vi "RS232RxDataFIFO.vi"   [LabVIEW 2016]
uses:
  <vilib>/rvi/Emulation/niFpgaGetClockAttributes.vi
  <vilib>/rvi/Emulation/niFpgaSctlEmulationGetInTimedLoop.vi
  <vilib>/rvi/Emulation/niFpgaEmulationReportErrorSimple.vi
  <vilib>/rvi/Emulation/niFpgaEmulationIsFPGAContextNoSignature.vi
  <vilib>/rvi/FIFO/Fifo_Resource/nirvififoEmulationSetSize.vi
  <vilib>/rvi/DataTransferAndStorage/Container/Common/niFpgaContainerGetUniqueNameForEmu.vi
  <vilib>/rvi/FIFO/Fifo_Resource/nirviFifoEmulationQueueMgr.vi
  <instcachedir>/0/nirviFifoEmulationQueueMgr_E5CAEC123FF24DC58D834DCA3CDAA9B5.lvgen/nirviFifoEmulationQueueMgr_E5CAEC123FF24DC58D834DCA3CDAA9B5_009.vi
  <vilib>/rvi/Emulation/niFpgaProcessEmulError.vi
  <vilib>/rvi/interface/RandomDataEmulation/niFpgaRandomDataHandleErrors.vi
  <vilib>/rvi/errors/niFpgaSetErrorForExecOnDevCompSimple.vi
  <vilib>/rvi/eio/common/nirviEmuReportErrorAndStop.vi
  <vilib>/Utility/error.llb/Clear Errors.vi
  <vilib>/rvi/FIFO/Fifo_Resource/nirvififoEmulationCreateLock.vi
  <vilib>/rvi/FIFO/Fifo_Resource/nirvififoEmulationObtainLock.vi
  <vilib>/rvi/FIFO/Fifo_Resource/nirvififoEmulationReleaseLock.vi
  <vilib>/rvi/occurrence/nirviWaitOnOccurrenceBase.vi
  <vilib>/rvi/errors/nirviReportUnexpectedCaseInternalError.vi
  <vilib>/rvi/errors/nirviReportUnexpectedCaseInternalError (U32).vi
  <vilib>/rvi/Emulation/niFpgaCriticalErrorInLSC.vi
  <vilib>/rvi/DataTransferAndStorage/Container/XNode/niFpgaContainer.xnode
  <vilib>/rvi/FIFO/Fifo_Resource/nirvififoEmulationGetNumberOfElementsToRead.vi
  <vilib>/rvi/interface/RandomDataEmulation/nirviRandomDataFpgaReadWriteTemplate.vi
  <vilib>/rvi/FIFO/Fifo_Resource/nirvififoEmulationRead.vi
  Common_FPGA_FIFO/FPGAFIFO.lvlib
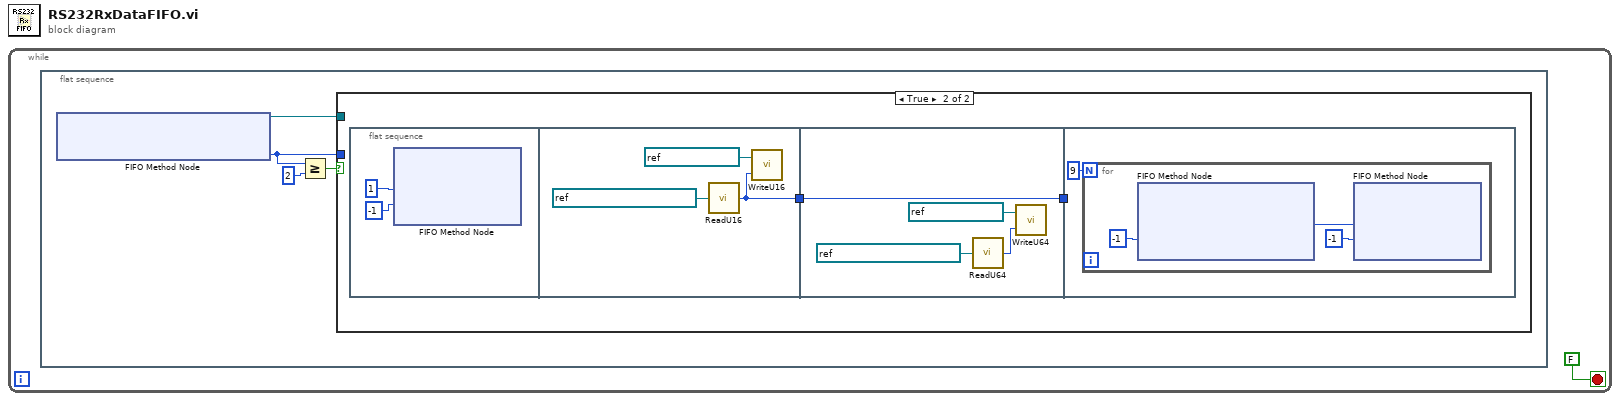
[diagram p0: block diagram]
diagram:
  n1 = while {
    stop <- FALSE stop-if-true
    n2 = flat-sequence {
      frame #0 {
        n3 = xnode ("FIFO Method Node")() -> ("Number of Elements to Read"=w2:u32, "FIFO Out"=w3:refnum<k21>)  [unwired: 1 in]
        n4 = Greater Or Equal?(x=w2, y=u32 2) -> (x >= y?=w4:bool)
        n5 = case shown="True" w4 {
          tunnel: w3 -> [_ _]
          tunnel: w2 -> [_ _]
          frame False {
          }
          frame True {
            n6 = flat-sequence {
              tunnel: [w10] -> w6
              tunnel: [w13] -> w7
              tunnel: w6 -> [w13]
              tunnel: w7 -> [_]
              frame #0 {
                n7 = xnode ("FIFO Method Node")("Element"=u8 1, "Timeout"=-1) -> ()  [unwired: 1 in, 2 out]
              }
              frame #1 {
                n8 = call "ReadU16.vi"("FIFO"=refnum<k21> "T7InclinometerRxFIFO") -> ("U16"=w10:u16)
                n9 = call "WriteU16.vi"("U16"=w10, "FIFO"=refnum<k21> "RS232RxFIFO") -> ()  [unwired: 1 in]
              }
              frame #2 {
                n10 = call "ReadU64.vi"("FIFO"=refnum<k21> "T7InclinometerRxFIFO") -> ("U64"=w14:u64)
                n11 = call "WriteU64.vi"("U64"=w14, "FIFO"=refnum<k21> "RS232RxFIFO") -> ()  [unwired: 1 in]
              }
              frame #3 {
                n12 = for {
                  N: 9 -> [_]
                  n13 = xnode ("FIFO Method Node")("Timeout"=-1) -> ("Element"=w18:u8)  [unwired: 1 in, 2 out]
                  n14 = xnode ("FIFO Method Node")("Element"=w18, "Timeout"=-1) -> ()  [unwired: 1 in, 2 out]
                }
              }
            }
          }
        }
      }
    }
  }
